vi "From Variant.vi"(8 "Error In":errorcluster, 10 "Variant":variant, 11 "2D Bool In":refnum<class "2D Bool.lvclass">) -> (0 "Error Out":errorcluster, 3 "2D Bool Out":refnum<class "2D Bool.lvclass">)   [LabVIEW 2020, in "NI_VIAnCFGDataStructure.lvlib" / "2D Bool.lvclass"]
doc: "Dynamic dispatch interface for conversion of variant LV data to Tree Data classes."
uses:
  <vilib>/addons/analyzer/VIAnCFGDataStructure/Data Types/2D Bool/2D Bool.lvclass
  <vilib>/addons/analyzer/VIAnCFGDataStructure/Data Types/2D Bool/2D Bool.lvclass/2D Bool.ctl
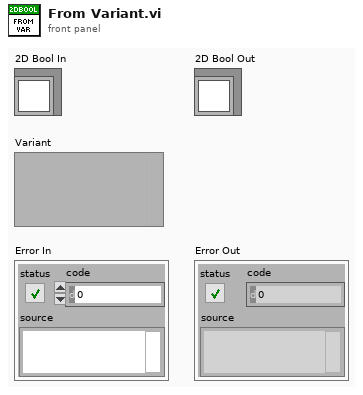
[diagram p1: front panel]
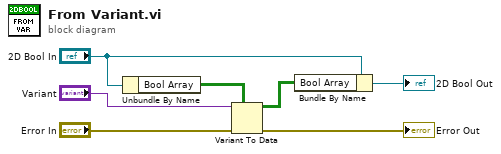
[diagram p0: block diagram]
diagram:
  n1 = Unbundle By Name("2D Bool In") -> ("Bool Array"=w5:bool[][])
  n2 = Variant To Data(error in="Error In", type=w5, Variant="Variant") -> (data=w3:bool[][], error out=→"Error Out":errorcluster)
  n3 = Bundle By Name(cluster="2D Bool In", "Bool Array"=w3) -> (→"2D Bool Out":refnum<class "2D Bool.lvclass">)
